vi "List this level build spec.vi"(8 "error in (no error)":errorcluster, 11 "project path":path) -> (0 "error out":errorcluster, 3 "Build Specs":T1(array[cluster]))   [LabVIEW 2019]
uses:
  <vilib>/xml/Close Reference(Node).vi
  <vilib>/xml/Load XML File.vi
  <vilib>/xml/NI_XML.lvlib
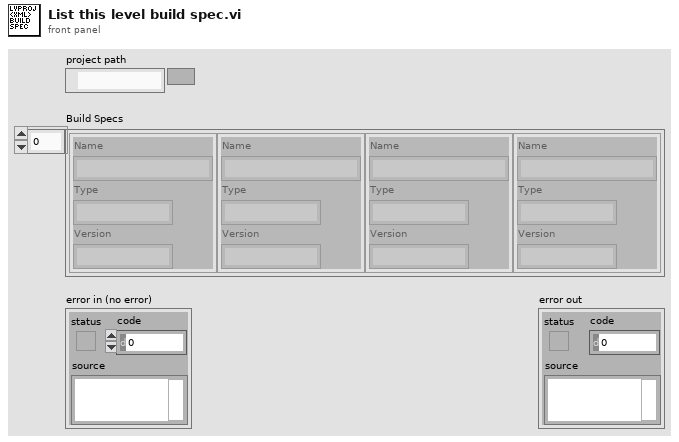
[diagram p1: front panel]
types:
  T1 = cluster{"Name":string, "Type":string, "Version":string}[]
  T2 = cluster{"Name":string, "Type":string, "Version":string}
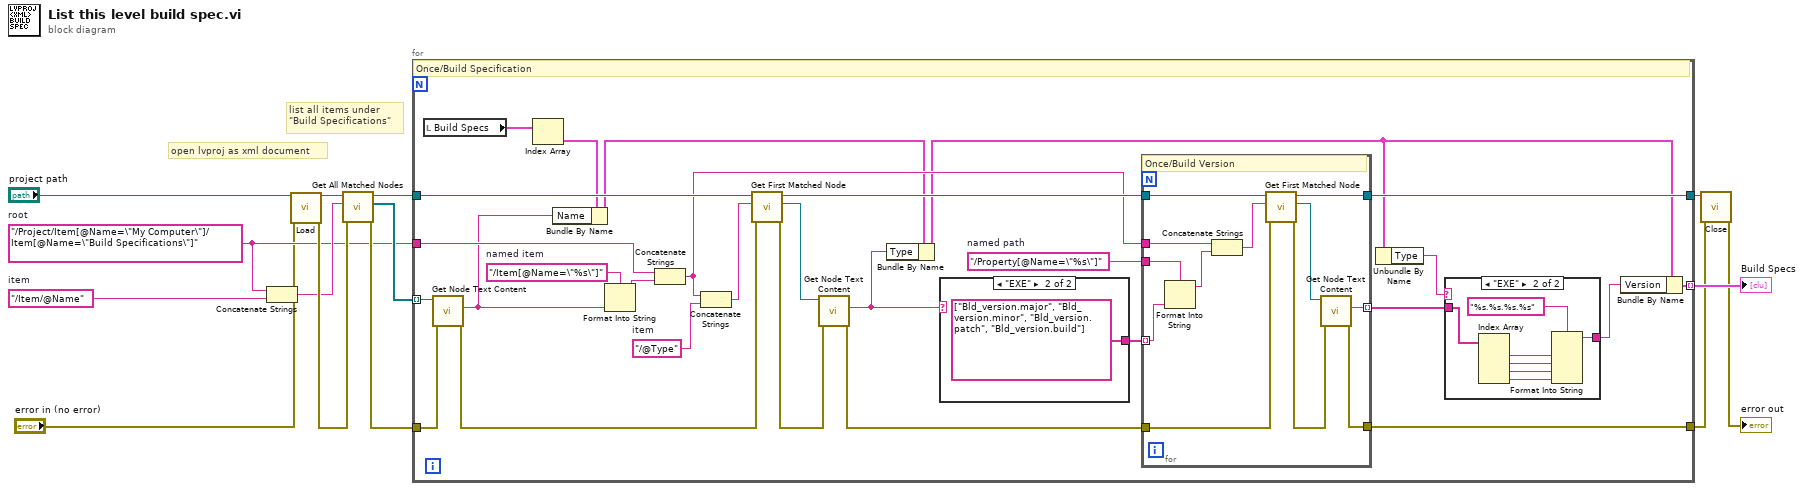
[diagram p0: block diagram]
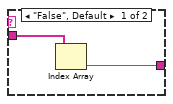
[diagram p2: hidden frame]
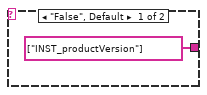
[diagram p3: hidden frame]
diagram:
  w7 = "/Item/@Name"  # item
  w5 = "/Project/Item[@Name=\"My Computer\"]/Item[@Name=\"Build Specifications\"]"  # root
  # "list all items under\n\"Build Specifications\""
  # "open lvproj as xml document"
  n1 = Concatenate Strings(w5, w7) -> (w6:string)
  n2 = call-poly <vilib>:"Load.vi"("path to XML document"="project path", "error in (no error)"="error in (no error)") -> ("DOM document out"=w12:refnum<k20>, "error out"=w11:errorcluster)  [unwired: 11 in, 1 out]
  n3 = call <vilib>:"Get All Matched Nodes.vi"("error in (no error)"=w11, "XPath expression"=w6, "node in"=w12) -> ("error out"=w8:errorcluster, "node result array"=w10:refnum<k20>[], "node out"=w9:refnum<k20>)  [unwired: 6 in]
  n4 = for {
    tunnel: w10 -> [w42] mode=indexing
    tunnel: w9 -> [w41]
    tunnel: w5 -> [w21]
    tunnel: w8 -> [w40]
    tunnel: [w25] -> w4
    tunnel: [w22] -> w13 mode=indexing
    tunnel: [w27] -> w3
    w31 = "/Property[@Name=\"%s\"]"  # named path
    w33 = "/@Type"  # item
    w35 = "/Item[@Name=\"%s\"]"  # named item
    # "Once/Build Specification"
    n5 = local read "Build Specs"() -> (w36:T1)
    n6 = call <vilib>:"Get Node Text Content.vi"("error in (no error)"=w40, "node in"=w42) -> ("error out"=w39:errorcluster, "node text"=w17:string)  [unwired: 7 in, 1 out]
    n7 = Index Array(array=w36) -> (element=w16:T2)  [unwired: 1 in]
    n8 = Bundle By Name(cluster=w16, "Name"=w17) -> (w15:T2)
    n9 = Format Into String(format string=w35, w17) -> (resulting string=w34:string)  [unwired: 2 in, 1 out]
    n10 = Concatenate Strings(w21, w34) -> (w26:string)
    n11 = Concatenate Strings(w26, w33) -> (w32:string)
    n12 = call <vilib>:"Get First Matched Node.vi"("error in (no error)"=w39, "XPath expression"=w32, "node in"=w41) -> ("error out"=w37:errorcluster, "node result"=w38:refnum<k20>, "node out"=w29:refnum<k20>)  [unwired: 6 in]
    n13 = call <vilib>:"Get Node Text Content.vi"("error in (no error)"=w37, "node in"=w38) -> ("error out"=w28:errorcluster, "node text"=w19:string)  [unwired: 7 in, 1 out]
    n14 = Bundle By Name(cluster=w15, "Type"=w19) -> (w20:T2)
    n15 = case shown="\"EXE\"" w19 {
      tunnel: [string[] ["INST_productVersion"] ("XPath expression") string[] ["Bld_version.major", "Bld_version.minor", "Bld_version.patch", "Bld_version.build"] ("XPath expression")] -> w30
      frame "False", Default {
      }
      frame "EXE" {
      }
    }
    n16 = for {
      tunnel: w31 -> [w54]
      tunnel: w30 -> [w53] mode=indexing
      tunnel: w29 -> [w48]
      tunnel: w28 -> [w47]
      tunnel: [w46] -> w27
      tunnel: w26 -> [w45]
      tunnel: [w44] -> w25
      tunnel: [w43] -> w24 mode=indexing
      # "Once/Build Version"
      n17 = Format Into String(format string=w54, w53) -> (resulting string=w51:string)  [unwired: 2 in, 1 out]
      n18 = Concatenate Strings(w45, w51) -> (w50:string)
      n19 = call <vilib>:"Get First Matched Node.vi"("error in (no error)"=w47, "XPath expression"=w50, "node in"=w48) -> ("error out"=w49:errorcluster, "node result"=w52:refnum<k20>, "node out"=w44:refnum<k20>)  [unwired: 6 in]
      n20 = call <vilib>:"Get Node Text Content.vi"("error in (no error)"=w49, "node in"=w52) -> ("error out"=w46:errorcluster, "node text"=w43:string)  [unwired: 7 in, 1 out]
    }
    n21 = Unbundle By Name(w20) -> ("Type"=w18:string)
    n22 = case shown="\"EXE\"" w18 {
      tunnel: w24 -> [w56 w62]
      tunnel: [w55 w57] -> w23
      frame "False", Default {
        n23 = Index Array(array=w56) -> (element=w55:string)  [unwired: 1 in]
      }
      frame "EXE" {
        n24 = Index Array(array=w62) -> (element #1=w61:string, element #2=w58:string, element #3=w59:string, element #4=w60:string)  [unwired: 4 in]
        n25 = Format Into String(format string="%s.%s.%s.%s", w61, w58, w59, w60) -> (resulting string=w57:string)  [unwired: 2 in, 1 out]
      }
    }
    n26 = Bundle By Name(cluster=w20, "Version"=w23) -> (w22:T2)
  }
  "Build Specs" <- w13
  n27 = call-poly <vilib>:"Close.vi"("error in (no error)"=w3, "node"=w4) -> ("error out"=→"error out":errorcluster)  [unwired: 7 in]
